vi "RT_Main_network_shared_variable_try.vi"() -> ()   [LabVIEW 2020]
uses:
  <vilib>/Platform/TimedLoop/XDataNode/timing_clust.ctl
  <vilib>/Platform/TimedLoop/XDataNode/nitl_modes.ctl
  <vilib>/Platform/TimedLoop/XDataNode/wakeup.ctl
  <vilib>/platform/TimedLoop/XDataNode/XDataNode.xnode
  <vilib>/Platform/TimedLoop/XDataNode/XDNodeRunTimeDep.lvlib
panel:
  out "Overflow":bool
  out "# elements in \nAI buffer":u32
  out "# elements  in \ncount FIFO":u32
  out "RT FIFO Analog Input\ntimed out? \n(red when bad)":bool
  out "RT FIFO Count\ntimed out? \n(red when bad)":bool
  out "Analog network\n writer time out":bool
  out "Count network\n writer time Out":bool
  # "RT FIFO Health"
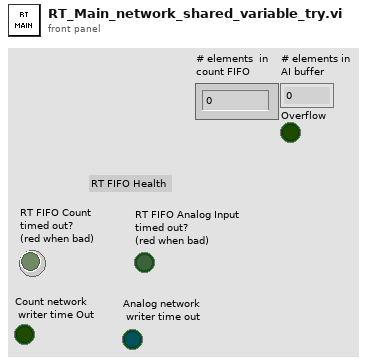
[diagram p1: front panel]
types:
  T1 = cluster{"Count RT FIFO":refnum<k33>, "Analog RT FIFO":refnum<k33>, "Analog Writer":refnum<k21>, "Count Writer":refnum<k21>}
  T2 = typedef "XDNodeRunTimeDep.lvlib/timing_clust.ctl" = cluster{"Expected End [f-1]":u64, "Actual End [f-1]":u64, "Finished Late? [f-1]":bool, "Expected End [i-1]":u64, "Actual End [i-1]":u64, "Finished Late? [i-1]":bool, "Expected Start [i]":u64, "Actual Start [i]":u64, "Expected Start [f]":u64, "Actual Start [f]":u64, "Source Name":string, "Structure Name":string, "Period":i64, "Deadline":i64, "Offset":i64, "Start":i64, "Priority":i32, "Timeout":i32, "Mode":T3, "Wakeup Reason":T4, "Error":errorcluster, "Source Type":string, "Secondary Source Type":string, "Global End Time":u64, "Global Start Time":u64, "Frame Duration":u64, "Iteration Duration":u64, "Assigned CPU":i32, "I/O Scan Engine Mode":u32}
  T3 = typedef "XDNodeRunTimeDep.lvlib/nitl_modes.ctl" = enum32{"No Change", "Process missed periods, maintain original phase", "Discard missed periods, maintain original phase", "Process missed periods, ignore original phase", "Discard missed periods, ignore original phase"}
  T4 = typedef "XDNodeRunTimeDep.lvlib/wakeup.ctl" = enum32{"Normal", "Aborted", "Asynchronous wakeup", "Timing source error", "Timed loop error", "Timeout"}
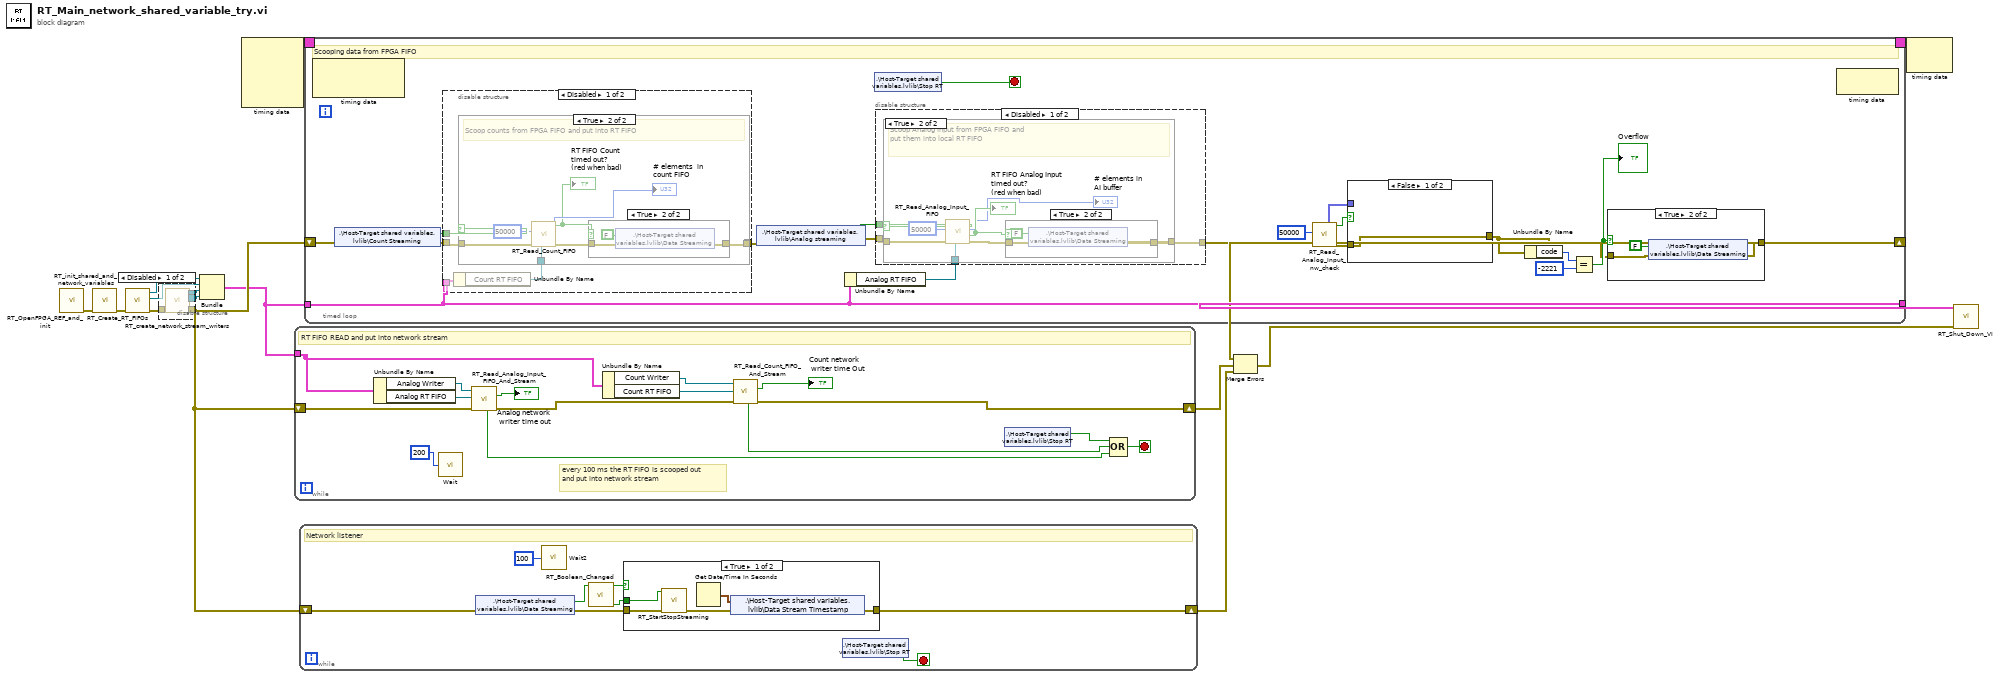
[diagram p0: block diagram]
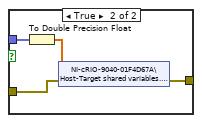
[diagram p5: hidden frame]
diagram:
  n1 = call "RT_OpenFPGA_REF_and_init.vi"() -> ("error out"=w15:errorcluster)  [unwired: 11 in]
  n2 = call "RT_init_shared_and_network_variables.vi"("error in (no error)"=w15) -> ("error out"=w16:errorcluster)  [unwired: 10 in]
  n3 = call "RT_Create_RT_FIFOs.vi"("error in (no error)"=w16) -> ("error out"=w12:errorcluster, "Analog RT FIFO"=w9:refnum<k33>, "Count RT FIFO"=w10:refnum<k33>)  [unwired: 8 in]
  n4 = disable-structure shown="Disabled" {
    disable-tunnel: w12 -> [w20 _]
    disable-tunnel: [w19 _] -> w11
    disable-tunnel: [w18 _] -> w8
    disable-tunnel: [w17 _] -> w7
    frame Disabled {
      n5 = call "RT_create_network_stream_writers.vi"("error in (no error)"=w20) -> ("error out"=w19:errorcluster, "Count Writer"=w17:refnum<k21>, "Analog Writer"=w18:refnum<k21>)  [unwired: 8 in]
    }
    frame Enabled {
    }
  }
  n6 = Bundle("Count RT FIFO"=w10, "Analog RT FIFO"=w9, "Analog Writer"=w8, "Count Writer"=w7) -> (w6:T1)  [unwired: 1 in]
  n7 = node-c288() -> (w14:T2)  [unwired: 4 in]
  n8 = while {
    shift-right: [w31] -> w3
    shift-left: w11 -> [w30]
    tunnel: w6 -> [w27]
    stop <- w33 stop-if-true
    # "every 100 ms the RT FIFO is scooped out and put into network stream"
    # "RT FIFO READ and put into network stream"
    n9 = Unbundle By Name(w27) -> ("Analog Writer"=w29:refnum<k21>, "Analog RT FIFO"=w28:refnum<k33>)
    n10 = call "Wait"("Count(mSec)"=u32 200) -> ()  [unwired: 1 out]
    n11 = call "RT_Read_Analog_Input_FIFO_And_Stream.vi"("error in (no error)"=w30, "rt fifo"=w28, "Network Stream endpoint"=w29) -> ("error out"=w32:errorcluster, "Network Stream Timed Out"=→"Analog network\n writer time out":bool, "Error FIFO"=w23:bool)  [unwired: 5 in, 1 out]
    n12 = Unbundle By Name(w27) -> ("Count Writer"=w26:refnum<k21>, "Count RT FIFO"=w25:refnum<k33>)
    n13 = call "RT_Read_Count_FIFO_And_Stream.vi"("error in (no error)"=w32, 10:"Refnum in"=w25, 11:"Refnum in"=w26) -> ("error out"=w31:errorcluster, "Network stream\n timed out"=→"Count network\n writer time Out":bool, "RT FIFO errored"=w22:bool)  [unwired: 5 in, 1 out]
    n14 = shared-variable ".\\Host-Target shared variables.lvlib\\Stop RT"() -> (w34:bool)  [unwired: 1 in, 1 out]
    n15 = Compound Arithmetic op=OR(w34, w22, w23) -> (w33:bool)
  }
  n16 = while {
    shift-right: [w37] -> w2
    shift-left: w11 -> [w38]
    stop <- w43 stop-if-true
    # "Network listener"
    n17 = shared-variable ".\\Host-Target shared variables.lvlib\\Data Streaming"(error in=w38) -> (w40:bool, error out=w39:errorcluster)
    n18 = call "Wait2"("Count(mSec)"=u32 100) -> ()  [unwired: 1 out]
    n19 = call "RT_Boolean_Changed.vi"("Boolean in"=w40) -> ("Value"=w36:bool, "Changed?"=w42:bool)  [unwired: 9 in]
    n20 = case shown="True" w42 {
      tunnel: w39 -> [w48 w49]
      tunnel: [w46 w49] -> w37
      tunnel: w36 -> [w44 _]
      frame True {
        n21 = call "RT_StartStopStreaming.vi"("error in (no error)"=w48, "Start/Stop?"=w44) -> ("error out"=w47:errorcluster)  [unwired: 9 in]
        n22 = Get Date/Time In Seconds() -> (seconds since 1Jan1904=w45:timestamp)
        n23 = shared-variable ".\\Host-Target shared variables.lvlib\\Data Stream Timestamp"(w45, error in=w47) -> (error out=w46:errorcluster)
      }
      frame False {
      }
    }
    n24 = shared-variable ".\\Host-Target shared variables.lvlib\\Stop RT"() -> (w43:bool)  [unwired: 1 in, 1 out]
  }
  n25 = timed-loop {
    timing: w14 -> [_]
    timing-out: [_] -> w13
    shift-right: [w50] -> w4
    shift-left: w11 -> [w62]
    tunnel: w6 -> [w61]
    tunnel: [w61] -> w5
    stop <- w64 stop-if-true
    # "Scooping data from FPGA FIFO"
    n26 = node-c288() -> ()  [unwired: 1 in, 2 out]
    n27 = shared-variable ".\\Host-Target shared variables.lvlib\\Count Streaming"(error in=w62) -> (w66:bool, error out=w67:errorcluster)
    n28 = disable-structure shown="Disabled" {
      disable-tunnel: w67 -> [w98 w111]
      disable-tunnel: w66 -> [w97 _]
      disable-tunnel: [w96 w111] -> w63
      disable-tunnel: w61 -> [w94 _]
      frame Disabled {
        n29 = Unbundle By Name(w94) -> ("Count RT FIFO"=w95:refnum<k33>)
        n30 = case shown="True" w97 {
          tunnel: w98 -> [w99 w106]
          tunnel: [w99 w103] -> w96
          tunnel: w95 -> [_ w102]
          frame False {
          }
          frame True {
            # "Scoop counts from FPGA FIFO and put into RT FIFO"
            n31 = call "RT_Read_Count_FIFO.vi"("rt fifo"=w102, "error in (no error)"=w106, "Elements to read"=u32 50000) -> ("error out"=w105:errorcluster, "# elements 2"=→"# elements  in \ncount FIFO":u32, "timed out?"=w100:bool)  [unwired: 5 in, 1 out]
            "RT FIFO Count\ntimed out? \n(red when bad)" <- w100
            n32 = case shown="True" w100 {
              tunnel: w105 -> [w107 w110]
              tunnel: [w107 w109] -> w103
              frame False {
              }
              frame True {
                n33 = shared-variable ".\\Host-Target shared variables.lvlib\\Data Streaming"(FALSE ("Data Streaming"), error in=w110) -> (error out=w109:errorcluster)
              }
            }
          }
        }
      }
      frame Enabled {
      }
    }
    n34 = shared-variable ".\\Host-Target shared variables.lvlib\\Analog streaming"(error in=w63) -> (w65:bool, error out=w68:errorcluster)
    n35 = Unbundle By Name(w61) -> ("Analog RT FIFO"=w60:refnum<k33>)
    n36 = shared-variable ".\\Host-Target shared variables.lvlib\\Stop RT"() -> (w64:bool)  [unwired: 1 in, 1 out]
    n37 = disable-structure shown="Disabled" {
      disable-tunnel: w68 -> [w81 _]
      disable-tunnel: w65 -> [w80 _]
      disable-tunnel: [w79 _] -> w59
      disable-tunnel: w60 -> [w78 _]
      frame Disabled {
        n38 = case shown="True" w80 {
          tunnel: w81 -> [w82 w89]
          tunnel: [w82 w88] -> w79
          tunnel: w78 -> [_ w85]
          frame False {
          }
          frame True {
            # "Scoop Analog Input from FPGA FIFO and\nput them into local RT FIFO"
            n39 = call "RT_Read_Analog_Input_FIFO.vi"("rt fifo"=w85, "error in (no error)"=w89, "Number Of Points"=u32 50000) -> ("error out"=w87:errorcluster, "timed out?"=w84:bool, "# elements"=→"# elements in \nAI buffer":u32)  [unwired: 4 in, 2 out]
            "RT FIFO Analog Input\ntimed out? \n(red when bad)" <- w84
            n40 = case shown="True" w84 {
              tunnel: [w90 w93] -> w88
              tunnel: w87 -> [w90 w92]
              frame False {
              }
              frame True {
                n41 = shared-variable ".\\Host-Target shared variables.lvlib\\Data Streaming"(FALSE ("Data Streaming"), error in=w92) -> (error out=w93:errorcluster)
              }
            }
          }
        }
      }
      frame Enabled {
      }
    }
    n42 = call "RT_Read_Analog_Input_nw_check.vi"("error in (no error)"=w59, "Number Of Points"=u32 50000) -> ("error out"=w55:errorcluster, "data read"=w57:bool, "Data"=w56:fxp<+/-,17,5>[])  [unwired: 7 in]
    n43 = case shown="False" w57 {
      tunnel: w56 -> [_ w77]
      tunnel: w55 -> [w73 w75]
      tunnel: [w73 w74] -> w51
      frame False {
      }
      frame True {
        n44 = To Double Precision Float(number=w77) -> (double precision float=w76:dbl[])
        n45 = shared-variable "NI-cRIO-9040-01F4D67A\\Host-Target shared variables.lvlib\\AnalogInput"(w76, error in=w75) -> (error out=w74:errorcluster)
      }
    }
    n46 = Unbundle By Name(w51) -> ("code"=w54:i32)
    n47 = Equal?(x=w54, y=-2221) -> (x = y?=w52:bool)
    "Overflow" <- w52
    n48 = case shown="True" w52 {
      tunnel: w51 -> [w69 w71]
      tunnel: [w69 w70] -> w50
      frame False {
      }
      frame True {
        n49 = shared-variable ".\\Host-Target shared variables.lvlib\\Data Streaming"(FALSE ("Data Streaming"), error in=w71) -> (error out=w70:errorcluster)
      }
    }
    n50 = node-c288() -> ()  [unwired: 1 in, 1 out]
  }
  n51 = Merge Errors(w4, w3, w2) -> (w1:errorcluster)
  n52 = node-c288(w13) -> ()  [unwired: 1 out]
  n53 = call "RT_Shut_Down_VI.vi"("error in (no error)"=w1, "Cluster"=w5) -> ()  [unwired: 10 in]
